vi "unpack_miniUSB_pulseCheck_ACF.vi"(8 "error in (no error)":errorcluster, 11 "Binary Data in":string) -> (0 "error out":errorcluster, 3 "Data out":dbl[][](array[numeric]))   [LabVIEW 2013]
doc: "# #############################################################################\n# ATTENTION\n# #############################################################################\n#\n# This software is for guidance only. It is provided \"as is\".\n# It only aims at providing coding information to the customer in order for\n# them to save time. As a result no warranties, whether express, implied or\n# statutory, including, but not limited to implied warranties of\n# merchantability and fitness for a particular purpose apply to this software.\n# A·P·E Angewandte Physik und Elektronik GmbH shall not be held liable for any\n# direct, indirect or consequential damages with respect to any claims arising\n# from the content of such sourcecode and/or the use made by customers of the\n# coding information contained herein in connection with their products.\n#\n# File Version: 1.0\n#\n# Changelog:\n# 1.0 - Initial Version\n#\n# #############################################################################"
panel:
  out "ACF":cluster{dbl[], dbl[]}(graph)
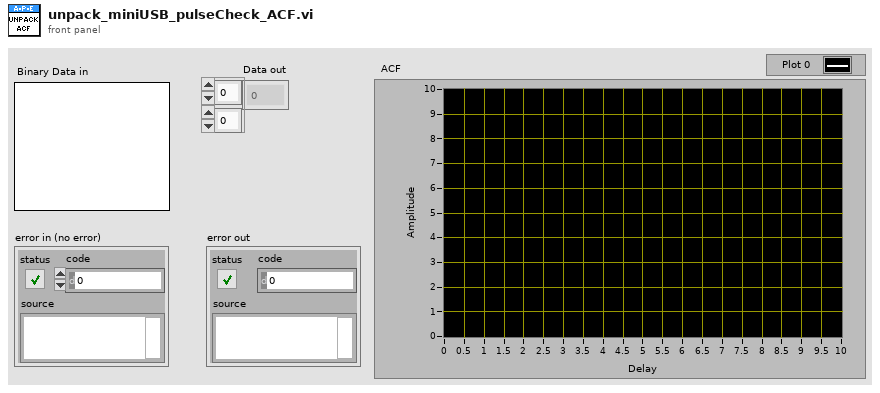
[diagram p1: front panel]
types:
  T1 = enum16{"big-endian, network order", "native, host order", "little-endian"}
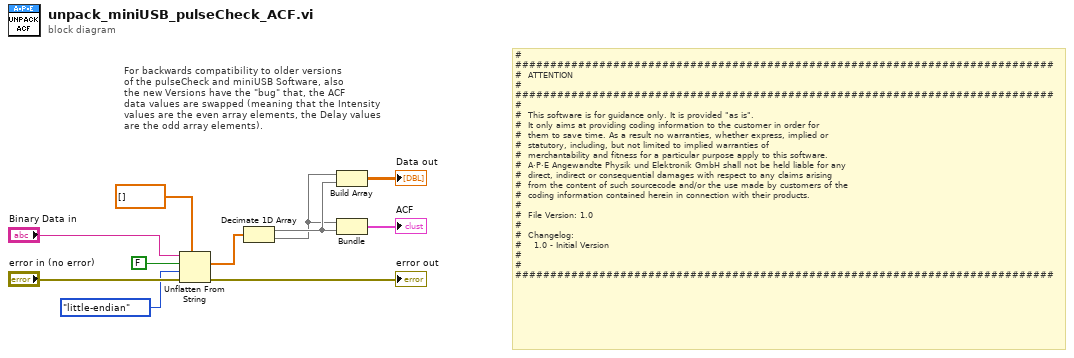
[diagram p0: block diagram]
diagram:
  # "# #############################################################################\n#  ATTENTION\n# #############################################################################\n#\n#  This software is for guidance only. It is provided \"as is\".\n#  It only aims at providing coding information to the customer in order for\n#  them to save time. As a result no warranties, whether express, implied or\n#  statutory, including, but not limited to implied warranties of\n#  merchantability and fitness for a particular purpose apply to this software.\n#  A·P·E Angewandte Physik und Elektronik GmbH shall not be held liable for any\n#  direct, indirect or consequential damages with respect to any claims arising\n#  from the content of such sourcecode and/or the use made by customers of the\n#  coding information contained herein in connection with their products.\n#\n#  File Version: 1.0\n#\n#  Changelog:\n#    1.0 - Initial Version\n#\n# #############################################################################"
  # "For backwards compatibility to older versions\nof the pulseCheck and miniUSB Software, also\nthe new Versions have the \"bug\" that, the ACF\ndata values are swapped (meaning that the Intensity\nvalues are the even array elements, the Delay values\nare the odd array elements)."
  n1 = Unflatten From String(type=dbl[] [] ("Data out"), binary string="Binary Data in", data includes array or string size? (T)=FALSE, byte order (0:big-endian, network order)=T1."little-endian", error in (no error)="error in (no error)") -> (value=w7:dbl[], error out=→"error out":errorcluster)  [unwired: 1 out]
  n2 = Decimate 1D Array(w7) -> (w3:dbl[], w2:dbl[])
  n3 = Build Array(w2, w3) -> (→"Data out":dbl[][])
  n4 = Bundle(w2, w3) -> (→"ACF":cluster{dbl[], dbl[]})  [unwired: 1 in]
